vi "String Proper Name from comma.vi"(11 "String Value":string) -> (3 "delimited string":string)   [LabVIEW 2012]
uses:
  <userlib>/_OpenG.lib/array/array.llb/Reorder 1D Array2 (String)__ogtk.vi
  <userlib>/_OpenG.lib/string/string.llb/Trim Whitespace (String)__ogtk.vi
  <userlib>/_OpenG.lib/string/string.llb/To Proper Case (String)__ogtk.vi
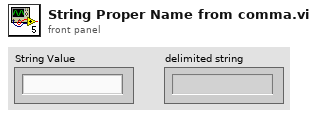
[diagram p1: front panel]
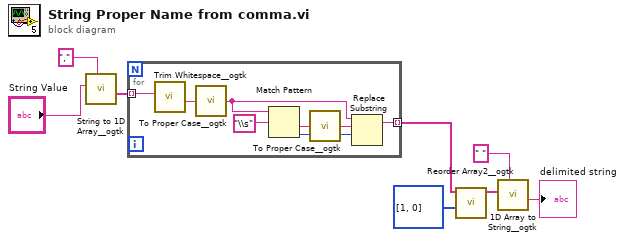
[diagram p0: block diagram]
diagram:
  n1 = call <userlib>:"String to 1D Array__ogtk.vi"("delimiter (Tab)"=",", "string"="String Value") -> ("Array of Strings"=w6:string[])  [unwired: 9 in]
  n2 = for {
    tunnel: w6 -> [w16] mode=indexing
    tunnel: [w9] -> w7 mode=indexing
    n3 = call-poly <userlib>:"Trim Whitespace__ogtk.vi"("String in"=w16) -> ("String out"=w15:string)  [unwired: 6 in]
    n4 = call-poly <userlib>:"To Proper Case__ogtk.vi"("string"=w15) -> ("proper case string"=w13:string)  [unwired: 4 in]
    n5 = Match Pattern(string=w13, regular expression="\\s") -> (after substring=w11:string, offset past match=w12:i32)  [unwired: 1 in, 2 out]
    n6 = call-poly <userlib>:"To Proper Case__ogtk.vi"("string"=w11) -> ("proper case string"=w10:string)  [unwired: 4 in]
    n7 = Replace Substring(3:w12, 4:w10, 5:w13) -> (1:w9:string)  [unwired: 1 in, 1 out]
  }
  n8 = call-poly <userlib>:"Reorder Array2__ogtk.vi"("indices"=i32[] [1, 0], "array"=w7) -> ("reordered array"=w5:string[])  [unwired: 9 in]
  n9 = call <userlib>:"1D Array to String__ogtk.vi"("delimiter (Tab)"=" ", "Array of Strings"=w5) -> ("delimited string"=→"delimited string":string)  [unwired: 9 in]
